vi "Dis- or en- able controls.vi"(8 "error in":errorcluster, 10 "Disabled":T1(ring), 11 "Control referencies":refnum<vi>[](array[refnum])) -> (0 "error out":errorcluster)   [LabVIEW 2021, in "MatS Libs.lvlib"]
uses:
  <userlib>/MatS Libs/MatS Libs.lvlib
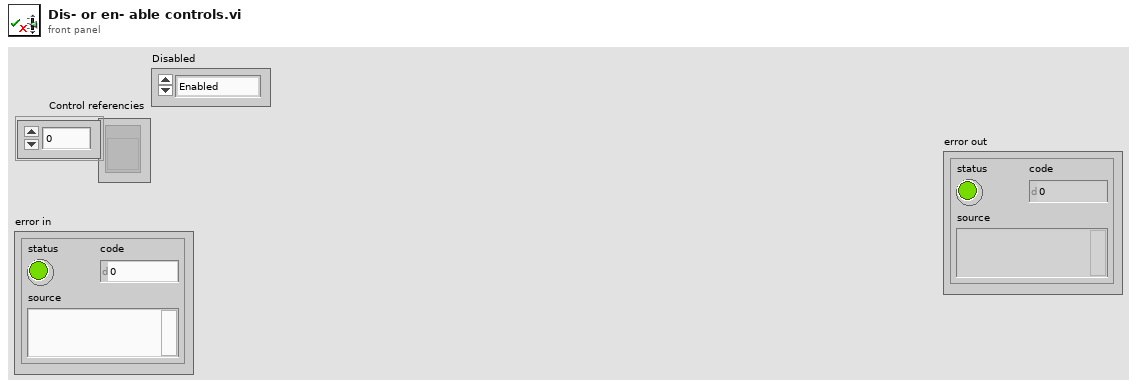
[diagram p1: front panel]
types:
  T1 = enum8{"Enabled", "Disabled", "Disabled and Grayed Out"}
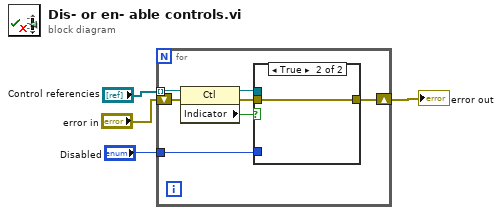
[diagram p0: block diagram]
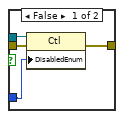
[diagram p2: hidden frame]
diagram:
  n1 = for {
    tunnel: "Control referencies" -> [w11] mode=indexing
    shift-right: [w10] -> w3
    shift-left: "error in" -> [w8]
    tunnel: "Disabled" -> [w5]
    n2 = property class="Ctl"(reference=w11, error in=w8) -> (reference out=w9:refnum<vi>, error out=w7:errorcluster, "Indicator"=w6:bool)
    n3 = case shown="True" w6 {
      tunnel: [w15 w16] -> w10
      tunnel: w9 -> [w14 _]
      tunnel: w7 -> [w13 w16]
      tunnel: w5 -> [w12 _]
      frame False {
        n4 = property class="Ctl"(reference=w14, error in=w13, "DisabledEnum"=w12) -> (error out=w15:errorcluster)  [unwired: 1 out]
      }
      frame True {
      }
    }
  }
  "error out" <- w3
